vi "GetSizeFactor.vi"(3 "error in (no error)":errorcluster, 5 "IMAQImage":T1) -> (0 "error out":errorcluster, 1 "Size factor":dbl, 2 "IMAQImage 2":T1)   [LabVIEW 2015]
uses:
  <vilib>/vision/Image Controls.llb/IMAQ Image.ctl
  <resource>/objmgr/IMAQImage.rc
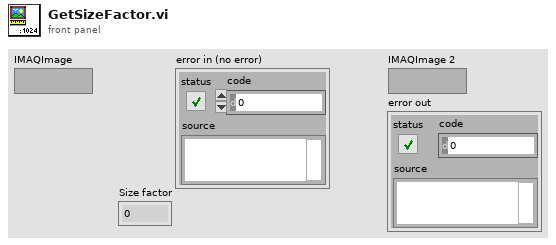
[diagram p1: front panel]
types:
  T1 = typedef "IMAQ Image.ctl" = refnum<image>
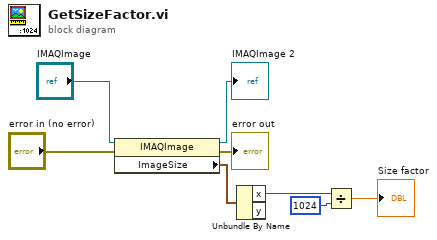
[diagram p0: block diagram]
diagram:
  n1 = property class="IMAQImage"(reference="IMAQImage", error in="error in (no error)") -> (reference out=→"IMAQImage 2":T1, error out=→"error out":errorcluster, "ImageSize"=w6:cluster{"x":i32, "y":i32})
  n2 = Unbundle By Name(w6) -> ("x"=w5:i32)  [unwired: 1 out]
  n3 = Divide(x=w5, y=u32 1024) -> (x/y=→"Size factor":dbl)
